vi "1D String To String.vi"(7 "Separate Sign":string=",", 10 "String Array In":string[](array[string])) -> (2 "String Out":string)   [LabVIEW 2024]
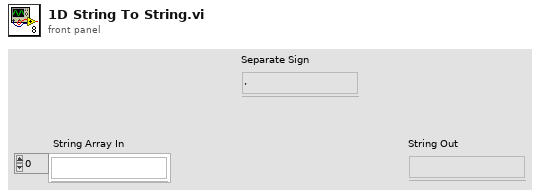
[diagram p1: front panel]
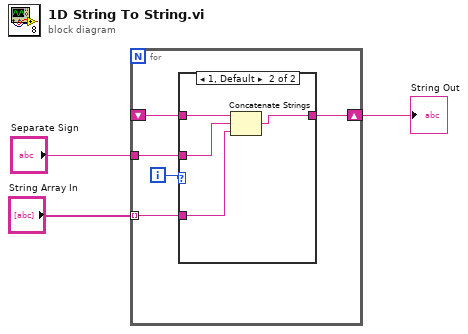
[diagram p0: block diagram]
diagram:
  n1 = for {
    tunnel: "String Array In" -> [w7] mode=indexing
    shift-right: [w6] -> w1
    shift-left: _ -> [w5]
    tunnel: "Separate Sign" -> [w4]
    i -> [w8]
    n2 = case shown="1, Default" w8 {
      tunnel: w7 -> [w9 w11]
      tunnel: [w9 w10] -> w6
      tunnel: w5 -> [_ w13]
      tunnel: w4 -> [_ w12]
      frame 0 {
      }
      frame 1, Default {
        n3 = Concatenate Strings(w13, w12, w11) -> (w10:string)
      }
    }
  }
  "String Out" <- w1
